vi "AI Loop.vi"() -> ()   [LabVIEW 2011]
uses:
  <vilib>/Platform/TimedLoop/XDataNode/timing_clust.ctl
  <vilib>/Platform/TimedLoop/XDataNode/nitl_modes.ctl
  <vilib>/Platform/TimedLoop/XDataNode/wakeup.ctl
  Utilities/Robot Parameters/Robot Parameters.vi
  <vilib>/Platform/TimedLoop/XDataNode/XDataNode.xnode
  <vilib>/Platform/TimedLoop/XDataNode/XDNodeRunTimeDep.lvlib
panel:
  in  "Direction":dbl[](array[numeric])
  in  "Magnitude":dbl[](array[numeric])
  in  "Line Data":T1(array[cluster])
  out "Outer threshold":dbl
  out "Inner threshold":dbl
  in  "Max speed (m/s)":dbl=0.5
  in  "No Occupancy":bool=TRUE
  out "Heading_Cmd":dbl
  out "VTan_Cmd":dbl
  out "VAng_Cmd":dbl
  out "Error Out":errorcluster
  in  "Error In":errorcluster
  in  "stop?":bool
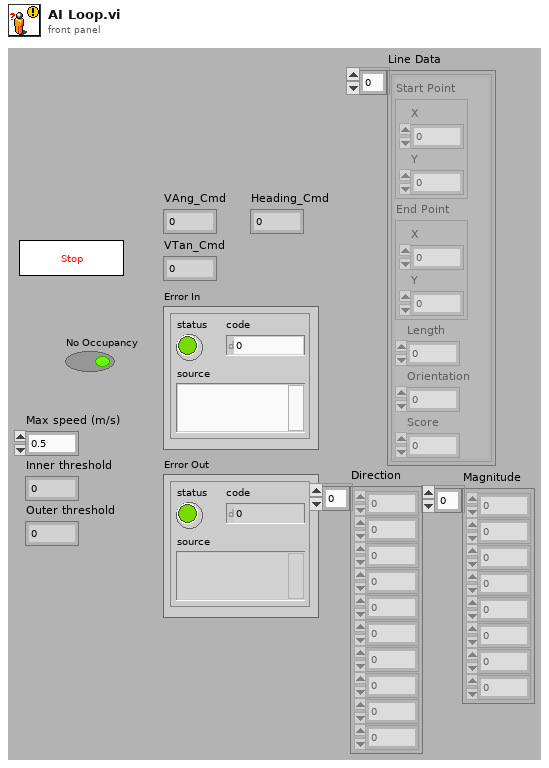
[diagram p1: front panel]
types:
  T1 = cluster{"Start Point":cluster{"X":sgl, "Y":sgl}, "End Point":cluster{"X":sgl, "Y":sgl}, "Length":dbl, "Orientation":dbl, "Score":dbl}[]
  T2 = enum16{"Idle", "Wiimote", "Joypad", "IGVC", "Avoide Objects", "Avoide Lines", "Path Planning", "Heading", "Waypoint"}
  T3 = typedef "XDNodeRunTimeDep.lvlib/timing_clust.ctl" = cluster{"Expected End [f-1]":u64, "Actual End [f-1]":u64, "Finished Late? [f-1]":bool, "Expected End [i-1]":u64, "Actual End [i-1]":u64, "Finished Late? [i-1]":bool, "Expected Start [i]":u64, "Actual Start [i]":u64, "Expected Start [f]":u64, "Actual Start [f]":u64, "Source Name":string, "Structure Name":string, "Period":i64, "Deadline":i64, "Offset":i64, "Start":i64, "Priority":i32, "Timeout":i32, "Mode":T4, "Wakeup Reason":T5, "Error":errorcluster, "Source Type":string, "Secondary Source Type":string, "Global End Time":u64, "Global Start Time":u64, "Frame Duration":u64, "Iteration Duration":u64, "Assigned CPU":i32, "I/O Scan Engine Mode":u32}
  T4 = typedef "XDNodeRunTimeDep.lvlib/nitl_modes.ctl" = enum32{"No Change", "Process missed periods, maintain original phase", "Discard missed periods, maintain original phase", "Process missed periods, ignore original phase", "Discard missed periods, ignore original phase"}
  T5 = typedef "XDNodeRunTimeDep.lvlib/wakeup.ctl" = enum32{"Normal", "Aborted", "Asynchronous wakeup", "Timing source error", "Timed loop error", "Timeout"}
  T6 = cluster{"Max speed (m/s)":dbl, "Inner threshold":dbl, "Outer threshold":dbl, "Data (deg) (m)":dbl[][], "Initialize?":bool, "Distance (m)":dbl, "Obstacle clearance (m)":dbl, "Current heading (deg)":dbl}
  T7 = cluster{"Position":cluster{"Roll":dbl, "Pitch":dbl, "Yaw":dbl}, "Orientation Matrix":dbl[][], "Magnetic Field":cluster{"Z-Axis Magnetic Field":dbl, "Y-Axis Magnetic Field":dbl, "X-Axis Magnetic Field":dbl}, "Acceleration":cluster{"Z-Axis Acceleration":dbl, "Y-Axis Acceleration":dbl, "X-Axis Acceleration":dbl}, "Angular Rate":cluster{"X-Axis Angular Rate":dbl, "Y-Axis Angular Rate":dbl, "Z-Axis Angular Rate":dbl}, "Quaternion":dbl[]}
  T8 = cluster{"command heading (rad)":dbl, "command vy":dbl, "command vx":dbl, "mask out":bool[], "command heading (deg)":dbl, "histogram out":dbl[]}
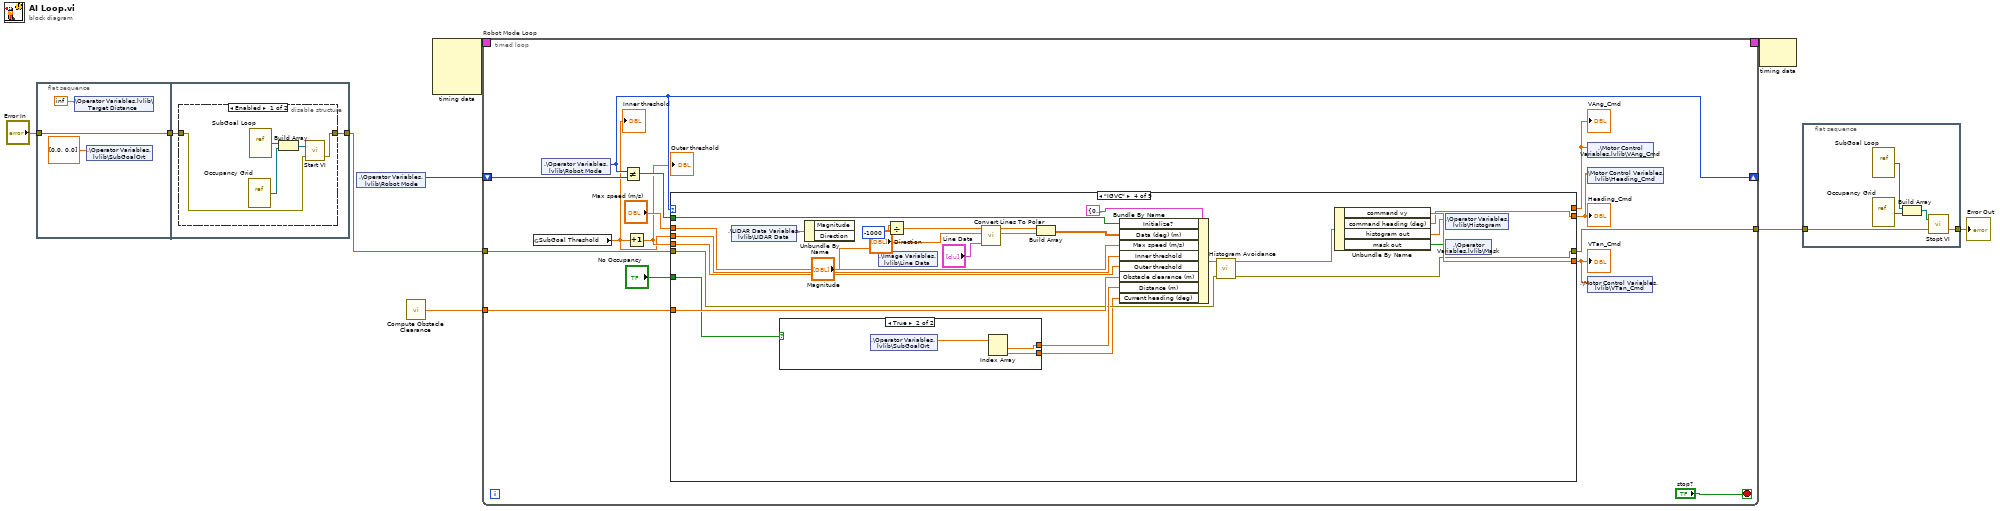
[diagram p0: block diagram]
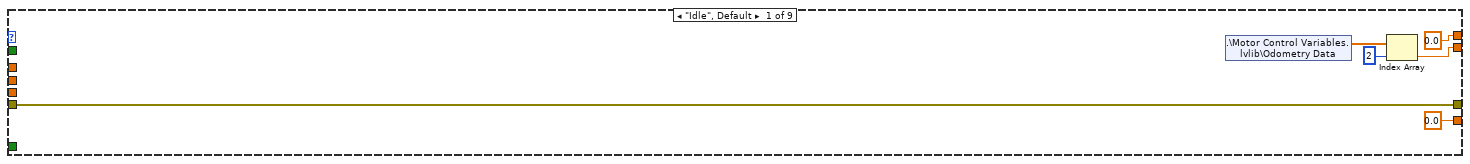
[diagram p3: hidden frame]
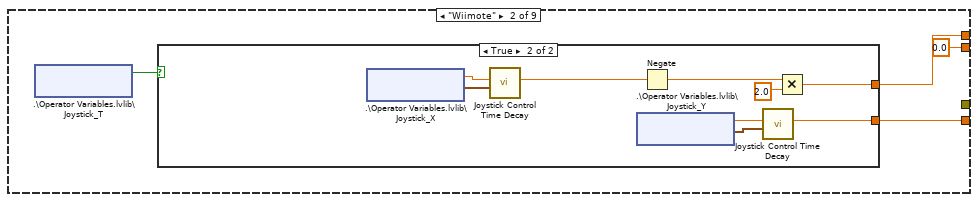
[diagram p4: hidden frame]
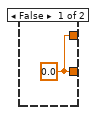
[diagram p5: hidden frame]
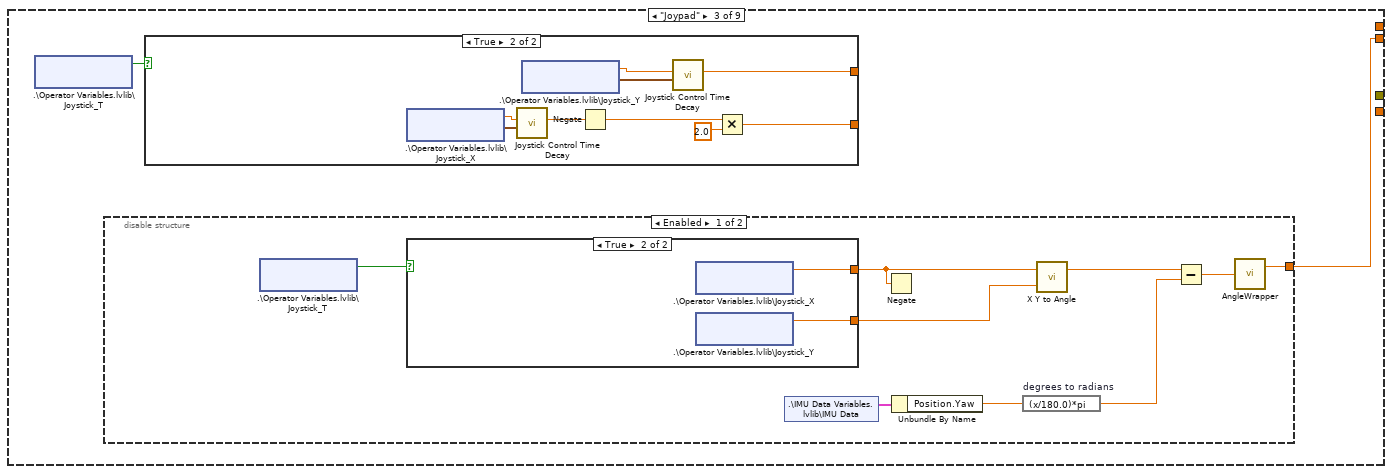
[diagram p6: hidden frame]
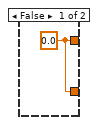
[diagram p7: hidden frame]
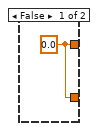
[diagram p9: hidden frame]
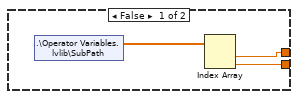
[diagram p10: hidden frame]
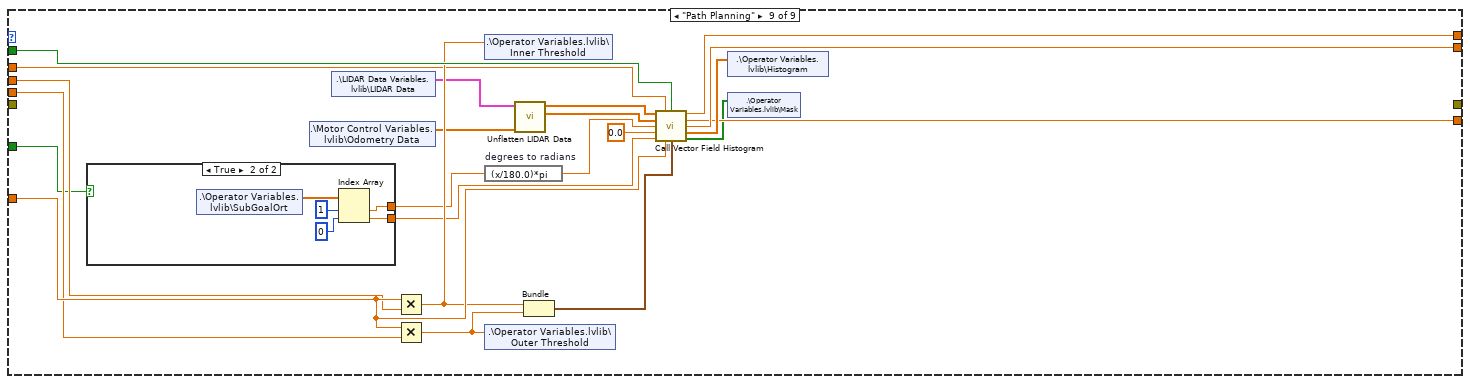
[diagram p15: hidden frame]
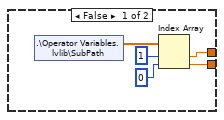
[diagram p16: hidden frame]
diagram:
  n1 = flat-sequence {
    tunnel: "Error In" -> [w11]
    tunnel: [w11] -> w4
    tunnel: [w13] -> w5
    tunnel: w4 -> [w14]
    frame #0 {
      n2 = shared-variable ".\\Operator Variables.lvlib\\Target Distance"(inf) -> ()  [unwired: 1 in, 1 out]
      n3 = shared-variable ".\\Operator Variables.lvlib\\SubGoalOrt"(dbl[] [0.0, 0.0] ("SubGoalOrt")) -> ()  [unwired: 1 in, 1 out]
    }
    frame #1 {
      n4 = disable-structure shown="Enabled" {
        disable-tunnel: w14 -> [w17 w20]
        disable-tunnel: [w16 w20] -> w13
        frame Enabled {
          n5 = vi-ref "Occupancy Grid.vi"() -> (w19:refnum<vi>)
          n6 = vi-ref "SubGoal Loop.vi"() -> (w15:refnum<vi>)
          n7 = Build Array(w15, w19) -> (w18:refnum<vi>[])
          n8 = call "Start VI.vi"("error in"=w17, "VI refnum"=w18) -> ("error out"=w16:errorcluster)  [unwired: 1 in]
        }
        frame Disabled {
        }
      }
    }
  }
  n9 = shared-variable ".\\Operator Variables.lvlib\\Robot Mode"() -> (w7:T2)  [unwired: 1 in, 1 out]
  n10 = call "Compute Obstacle Clearance.vi"() -> ("obstacle clearance (m)"=w1:dbl)  [unwired: 1 in]
  n11 = node-c288() -> (w9:T3)  [unwired: 4 in]
  n12 = timed-loop "Robot Mode Loop" {
    timing: w9 -> [_]
    timing-out: [_] -> w8
    tunnel: w1 -> [w34]
    shift-right: [w31] -> _
    shift-left: w7 -> [w32]
    tunnel: w5 -> [w24]
    tunnel: [w23] -> w2
    stop <- "stop?" stop-if-true
    n13 = global read "Robot Parameters.vi" "SubGoal Threshold"() -> (w21:dbl)
    "Inner threshold" <- w21
    n14 = shared-variable ".\\Operator Variables.lvlib\\Robot Mode"() -> (w31:T2)  [unwired: 1 in, 1 out]
    n15 = Not Equal?(x=w31, y=w32) -> (x != y?=w33:bool)
    n16 = Increment(x=w21) -> (x+1=w22:dbl)
    "Outer threshold" <- w22
    n17 = case shown="\"IGVC\"" w31 {
      tunnel: w34 -> [_ _ _ w97 _ _ _ _ w128]
      tunnel: [w36 0.0 ("command vy") w55 w92 _ _ _ _ w127] -> w30
      tunnel: [0.0 ("Double") w42 _ w93 _ _ _ _ w122] -> w29
      tunnel: [0.0 w41 _ _ _ _ _ _ w123] -> w28
      tunnel: w33 -> [_ _ _ w98 _ _ _ _ w130]
      tunnel: w21 -> [_ _ _ w101 _ _ _ _ w114]
      tunnel: w22 -> [_ _ _ w100 _ _ _ _ w113]
      tunnel: "Max speed (m/s)" -> [_ _ _ w102 _ _ _ _ w112]
      tunnel: "No Occupancy" -> [_ _ _ w96 _ _ _ _ w111]
      tunnel: w24 -> [w35 _ _ w89 _ _ _ _ _]
      tunnel: [w35 _ _ w88 _ _ _ _ _] -> w23
      frame "Idle", Default {
        n18 = shared-variable ".\\Motor Control Variables.lvlib\\Odometry Data"() -> (w38:dbl[])  [unwired: 1 in, 1 out]
        n19 = Index Array(array=w38, index=2) -> (element=w36:dbl)
      }
      frame "Wiimote" {
        n20 = shared-variable ".\\Operator Variables.lvlib\\Joystick_T"() -> (w44:bool)  [unwired: 1 in, 2 out]
        n21 = case shown="True" w44 {
          tunnel: [w45 w50] -> w42
          tunnel: [w45 w47] -> w41
          frame False {
            w45 = 0.0
          }
          frame True {
            n22 = shared-variable ".\\Operator Variables.lvlib\\Joystick_X"() -> (w54:dbl, w53:timestamp)  [unwired: 1 in, 1 out]
            n23 = call "Joystick Control Time Decay.vi"("Value"=w54, "Time Stamp"=w53) -> ("Decayed Value"=w49:dbl)  [unwired: 8 in]
            n24 = shared-variable ".\\Operator Variables.lvlib\\Joystick_Y"() -> (w51:dbl, w52:timestamp)  [unwired: 1 in, 1 out]
            n25 = Negate(x=w49) -> (-x=w48:dbl)
            n26 = call "Joystick Control Time Decay.vi"("Value"=w51, "Time Stamp"=w52) -> ("Decayed Value"=w50:dbl)  [unwired: 8 in]
            n27 = Multiply(x=w48, y=2.0) -> (x*y=w47:dbl)
          }
        }
      }
      frame "Joypad" {
        n28 = shared-variable ".\\Operator Variables.lvlib\\Joystick_T"() -> (w56:bool)  [unwired: 1 in, 2 out]
        n29 = disable-structure shown="Enabled" {
          disable-tunnel: [w57 _] -> w55
          frame Enabled {
            n30 = shared-variable ".\\Operator Variables.lvlib\\Joystick_T"() -> (w65:bool)  [unwired: 1 in, 2 out]
            n31 = case shown="True" w65 {
              tunnel: [w66 w67] -> w62
              tunnel: [w66 w68] -> w63
              frame False {
                w66 = 0.0
              }
              frame True {
                n32 = shared-variable ".\\Operator Variables.lvlib\\Joystick_X"() -> (w68:dbl)  [unwired: 1 in, 2 out]
                n33 = shared-variable ".\\Operator Variables.lvlib\\Joystick_Y"() -> (w67:dbl)  [unwired: 1 in, 2 out]
              }
            }
            n34 = shared-variable ".\\IMU Data Variables.lvlib\\IMU Data"() -> (w64:T7)  [unwired: 1 in, 1 out]
            n35 = Negate(x=w63) -> ()  [unwired: 1 out]
            n36 = Unbundle By Name(w64) -> ("Position.Yaw"=w61:dbl)
            n37 = expression code="(x/180.0)*pi" "degrees to radians"(w61) -> (w60:dbl)
            n38 = call "X Y to Angle.vi"("y"=w62, "x"=w63) -> ("Heading Out (rad)"=w59:dbl)  [unwired: 1 out]
            n39 = Subtract(x=w59, y=w60) -> (x-y=w58:dbl)
            n40 = call "AngleWrapper.vi"("Heading In (rad)"=w58) -> ("Heading Out (rad)"=w57:dbl)  [unwired: 1 out]
          }
          frame Disabled {
          }
        }
        n41 = case shown="True" w56 {
          tunnel: [w69 w74] -> _
          tunnel: [w69 w71] -> _
          frame False {
            w69 = 0.0
          }
          frame True {
            n42 = shared-variable ".\\Operator Variables.lvlib\\Joystick_X"() -> (w78:dbl, w77:timestamp)  [unwired: 1 in, 1 out]
            n43 = call "Joystick Control Time Decay.vi"("Value"=w78, "Time Stamp"=w77) -> ("Decayed Value"=w73:dbl)  [unwired: 8 in]
            n44 = shared-variable ".\\Operator Variables.lvlib\\Joystick_Y"() -> (w75:dbl, w76:timestamp)  [unwired: 1 in, 1 out]
            n45 = Negate(x=w73) -> (-x=w72:dbl)
            n46 = call "Joystick Control Time Decay.vi"("Value"=w75, "Time Stamp"=w76) -> ("Decayed Value"=w74:dbl)  [unwired: 8 in]
            n47 = Multiply(x=w72, y=2.0) -> (x*y=w71:dbl)
          }
        }
      }
      frame "IGVC" {
        n48 = shared-variable ".\\LIDAR Data Variables.lvlib\\LIDAR Data"() -> (w99:cluster{"Magnitude":dbl[], "Direction":dbl[]})  [unwired: 1 in, 1 out]
        n49 = case shown="True" w96 {
          tunnel: [w106 w109] -> w95
          tunnel: [w105 w108] -> w86
          frame False {
            n50 = shared-variable ".\\Operator Variables.lvlib\\SubPath"() -> (w107:dbl[])  [unwired: 1 in, 1 out]
            n51 = Index Array(array=w107) -> (element #1=w106:dbl, element #2=w105:dbl)  [unwired: 2 in]
          }
          frame True {
            n52 = shared-variable ".\\Operator Variables.lvlib\\SubGoalOrt"() -> (w110:dbl[])  [unwired: 1 in, 1 out]
            n53 = Index Array(array=w110) -> (element #1=w109:dbl, element #2=w108:dbl)  [unwired: 2 in]
          }
        }
        n54 = Unbundle By Name(w99) -> ()  [unwired: 2 out]
        n55 = shared-variable ".\\Image Variables.lvlib\\Line Data"() -> ()  [unwired: 1 in, 2 out]
        n56 = Divide(x="Magnitude", y=-1000) -> (x/y=w84:dbl[])
        n57 = call "Convert Lines To Polar.vi"("Lines In"="Line Data", "Angle In"="Direction", "Range In"=w84) -> ("Angle Out"=w82:dbl[], "Range Out"=w83:dbl[])  [unwired: 7 in]
        n58 = Build Array(w83, w82) -> (w85:dbl[][])
        n59 = Bundle By Name(cluster=T6 {"Max speed (m/s)"=0.4, "Inner threshold"=0.6, "Outer threshold"=1.1, "Data (deg) (m)"=[], "Initialize?"=FALSE, "Distance (m)"=0.0, "Obstacle clearance (m)"=1.0, "Current heading (deg)"=0.0} ("Control"), "Initialize?"=w98, "Data (deg) (m)"=w85, "Max speed (m/s)"=w102, "Inner threshold"=w101, "Outer threshold"=w100, "Obstacle clearance (m)"=w97, "Distance (m)"=w95, "Current heading (deg)"=w86) -> (w103:T6)
        n60 = call "Histogram Avoidance.vi"("Error In"=w89, "Control"=w103) -> ("Error Out"=w88:errorcluster, "Output"=w94:T8)  [unwired: 8 in]
        n61 = Unbundle By Name(w94) -> ("command vy"=w93:dbl, "command heading (deg)"=w92:dbl, "histogram out"=w91:dbl[], "mask out"=w90:bool[])
        n62 = shared-variable ".\\Operator Variables.lvlib\\Histogram"(w91) -> ()  [unwired: 1 in, 1 out]
        n63 = shared-variable ".\\Operator Variables.lvlib\\Mask"(w90) -> ()  [unwired: 1 in, 1 out]
      }
      frame "Avoide Objects" {
      }
      frame "Avoide Lines" {
      }
      frame "Heading" {
      }
      frame "Waypoint" {
      }
      frame "Path Planning" {
        n64 = case shown="True" w111 {
          tunnel: [w135 w139] -> w116
          tunnel: [w134 w138] -> w117
          frame False {
            n65 = shared-variable ".\\Operator Variables.lvlib\\SubPath"() -> (w133:dbl[])  [unwired: 1 in, 1 out]
            n66 = Index Array(array=w133, index #1=1 ("index"), index #2=0 ("index")) -> (element #1=w135:dbl, element #2=w134:dbl)
          }
          frame True {
            n67 = shared-variable ".\\Operator Variables.lvlib\\SubGoalOrt"() -> (w142:dbl[])  [unwired: 1 in, 1 out]
            n68 = Index Array(array=w142, index #1=1 ("index"), index #2=0 ("index")) -> (element #1=w139:dbl, element #2=w138:dbl)
          }
        }
        n69 = shared-variable ".\\Motor Control Variables.lvlib\\Odometry Data"() -> (w120:dbl[])  [unwired: 1 in, 1 out]
        n70 = shared-variable ".\\LIDAR Data Variables.lvlib\\LIDAR Data"() -> (w121:cluster{"Magnitude":dbl[], "Direction":dbl[]})  [unwired: 1 in, 1 out]
        n71 = Multiply(x=w128, y=w114) -> (x*y=w126:dbl)
        n72 = Multiply(x=w128, y=w113) -> (x*y=w125:dbl)
        n73 = shared-variable ".\\Operator Variables.lvlib\\Inner Threshold"(w126) -> ()  [unwired: 1 in, 1 out]
        n74 = expression code="(x/180.0)*pi" "degrees to radians"(w116) -> (w115:dbl)
        n75 = shared-variable ".\\Operator Variables.lvlib\\Outer Threshold"(w125) -> ()  [unwired: 1 in, 1 out]
        n76 = call "Unflatten LIDAR Data.vi"("Odometry Data"=w120, "LIDAR Data"=w121) -> ("Bearing (rad)"=w131:dbl[], "Range (m)"=w132:dbl[])  [unwired: 8 in]
        n77 = Bundle(w126, w125) -> (w124:cluster{dbl, dbl})  [unwired: 1 in]
        n78 = call "Call Vector Field Histogram.vi"("LIDAR magn. (m)"=w132, "max speed"=w112, "Initialize?"=w130, "LIDAR angle (rad)"=w131, "current heading (rad)"=w115, "target heading (rad)"=0.0 ("current heading (rad)"), "target distance"=w117, "obstacle clearance (m)"=w128, "thresholds"=w124) -> ("command vx"=w123:dbl, "command vy"=w122:dbl, "command heading (rad)"=w127:dbl, "histogram out"=w129:dbl[], "mask out"=w119:bool[])  [unwired: 2 in]
        n79 = shared-variable ".\\Operator Variables.lvlib\\Histogram"(w129) -> ()  [unwired: 1 in, 1 out]
        n80 = shared-variable ".\\Operator Variables.lvlib\\Mask"(w119) -> ()  [unwired: 1 in, 1 out]
      }
    }
    "VAng_Cmd" <- w28
    "VTan_Cmd" <- w29
    "Heading_Cmd" <- w30
    n81 = shared-variable ".\\Motor Control Variables.lvlib\\VAng_Cmd"(w28) -> ()  [unwired: 1 in, 1 out]
    n82 = shared-variable ".\\Motor Control Variables.lvlib\\Heading_Cmd"(w30) -> ()  [unwired: 1 in, 1 out]
    n83 = shared-variable ".\\Motor Control Variables.lvlib\\VTan_Cmd"(w29) -> ()  [unwired: 1 in, 1 out]
  }
  n84 = node-c288(w8) -> ()  [unwired: 1 out]
  n85 = flat-sequence {
    tunnel: [w146] -> w3
    tunnel: w2 -> [w147]
    frame #0 {
      n86 = vi-ref "Occupancy Grid.vi"() -> (w148:refnum<vi>)
      n87 = vi-ref "SubGoal Loop.vi"() -> (w145:refnum<vi>)
      n88 = Build Array(w145, w148) -> (w149:refnum<vi>[])
      n89 = call "Stopt VI.vi"("error in"=w147, "VI refnum"=w149) -> ("error out"=w146:errorcluster)  [unwired: 1 in]
    }
  }
  "Error Out" <- w3
